vi "Shooter Turn.vi"(8 "Difference":dbl, 9 "Axis Value":dbl, 11 "Condition":bool) -> (3 "Turn Speed":dbl)   [LabVIEW 2012]
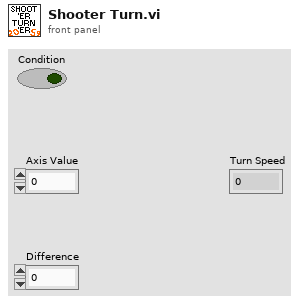
[diagram p1: front panel]
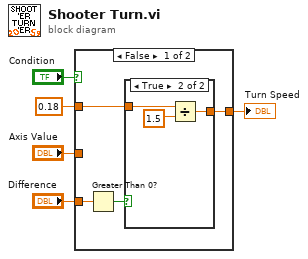
[diagram p0: block diagram]
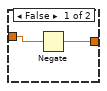
[diagram p2: hidden frame]
diagram:
  n1 = case shown="False" "Condition" {
    tunnel: [w7 w15] -> w1
    tunnel: "Axis Value" -> [_ w15]
    tunnel: 0.18 -> [w9 _]
    tunnel: "Difference" -> [w8 _]
    frame False {
      n2 = Greater Than 0?(x=w8) -> (x > 0?=w6:bool)
      n3 = case shown="True" w6 {
        tunnel: [w11 w14] -> w7
        tunnel: w9 -> [w10 w13]
        frame False {
          n4 = Negate(x=w10) -> (-x=w11:dbl)
        }
        frame True {
          n5 = Divide(x=w13, y=1.5) -> (x/y=w14:dbl)
        }
      }
    }
    frame True {
    }
  }
  "Turn Speed" <- w1
